vi "ImageUTMPosition.vi"(10 "Pixel Coordinates":cluster{"X":i32, "Y":i32}, 11 "MapDistanceInfo":T2 {"Top Left Pixel UTM"."North" format="%#_10f"; "Top Left Pixel UTM"."East" format="%#_8f"; "Bottom Right Pixel UTM"."North" format="%#_10f"; "Bottom Right Pixel UTM"."East" format="%#_8f"}) -> (3 "output cluster":T1 {"North" format="%#_10f"; "East" format="%#_8f"})   [LabVIEW 2013]
doc: "This VI takes a UTM position and information about an image (corner positions, m/pixel) and finds the pixel position of the UTM point."
uses:
  TypeDef/MapDistanceInfo.ctl
  cRIO_Code/Data/TypeDefs/UTM Location.ctl
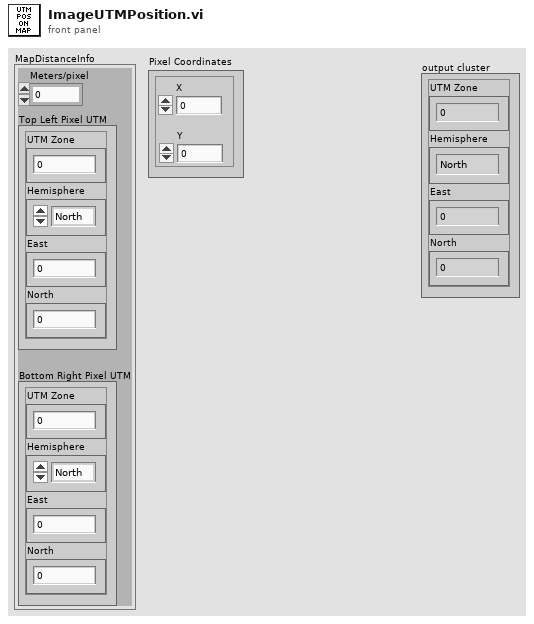
[diagram p1: front panel]
types:
  T1 = typedef "UTM Location.ctl" = cluster{"UTM Zone":dbl, "Hemisphere":enum16{"North", "South"}, "East":dbl, "North":dbl}
  T2 = typedef "MapDistanceInfo.ctl" = cluster{"Meters/pixel":dbl, "Top Left Pixel UTM":T1, "Bottom Right Pixel UTM":T1}
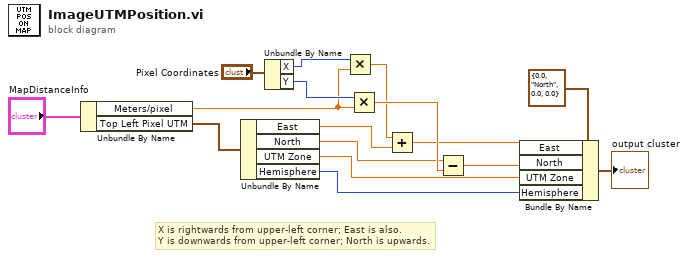
[diagram p0: block diagram]
diagram:
  # "X is rightwards from upper-left corner; East is also.\nY is downwards from upper-left corner; North is upwards."
  n1 = Unbundle By Name("MapDistanceInfo") -> ("Meters/pixel"=w7:dbl, "Top Left Pixel UTM"=w6:T1)
  n2 = Unbundle By Name(w6) -> ("East"=w4:dbl, "North"=w5:dbl, "UTM Zone"=w2:dbl, "Hemisphere"=w3:enum16{"North", "South"})
  n3 = Unbundle By Name("Pixel Coordinates") -> ("X"=w12:i32, "Y"=w11:i32)
  n4 = Multiply(x=w12, y=w7) -> (x*y=w15:dbl)
  n5 = Multiply(x=w11, y=w7) -> (x*y=w16:dbl)
  n6 = Add(x=w15, y=w4) -> (x+y=w14:dbl)
  n7 = Subtract(x=w5, y=w16) -> (x-y=w13:dbl)
  n8 = Bundle By Name(cluster=T1 {"UTM Zone"=0.0, "Hemisphere"=enum."North", "East"=0.0, "North"=0.0} ("UTM Location"), "East"=w14, "North"=w13, "UTM Zone"=w2, "Hemisphere"=w3) -> (→"output cluster":T1)
